vi "-8750 Error parsing BOOL from--error.vi"(8 "error in":errorcluster, 11 "String":string) -> (0 "error out":errorcluster)   [LabVIEW 2024, in "Config from XML.lvclass"]
uses:
  Config from XML.lvclass
  Config from XML.lvclass/Config from XML.ctl
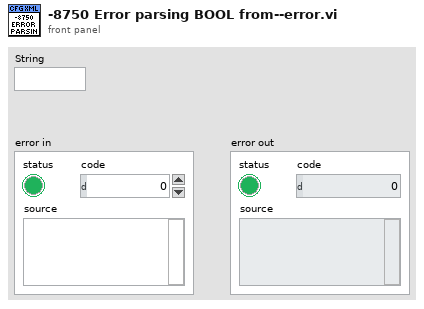
[diagram p1: front panel]
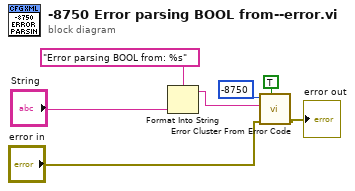
[diagram p0: block diagram]
diagram:
  n1 = Format Into String(format string="Error parsing BOOL from: %s", "String") -> (resulting string=w5:string)  [unwired: 2 in, 1 out]
  n2 = call <vilib>:"Error Cluster From Error Code.vi"("show call chain? (False)"=TRUE, "error in (no error)"="error in", "error message (\"\")"=w5, "error code (0)"=-8750) -> ("error out"=→"error out":errorcluster)  [unwired: 5 in]
